vi "Auto_Routine_QuickAuto.vi"(8 "error in (no error)":errorcluster, 9 "Distance(Back)":dbl, 10 "Game Piece":T1, 11 "Position":T2=enum."Middle") -> (0 "error out":errorcluster)   [LabVIEW 2020]
uses:
  Arm/ArmPositionPreset.ctl
  Arm/ArmGamePiecePreset.ctl
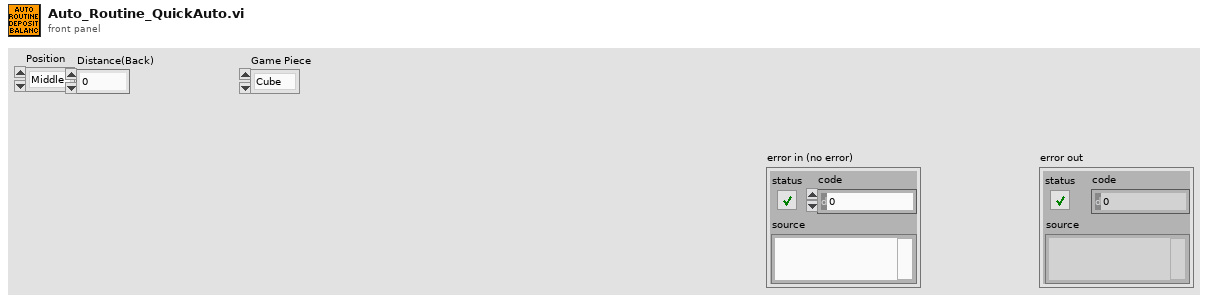
[diagram p1: front panel]
types:
  T1 = typedef "ArmGamePiecePreset.ctl" = enum16{"Cube", "Cone"}
  T2 = typedef "ArmPositionPreset.ctl" = enum16{"Upper", "Lower", "Middle", "Home", "Shelf", "Floor"}
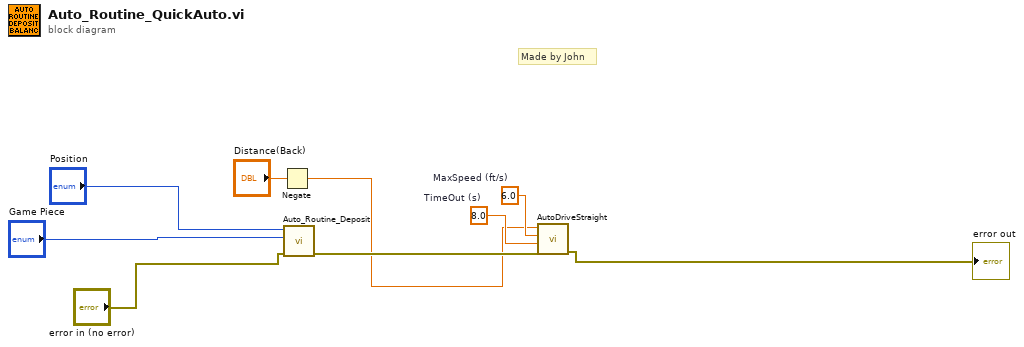
[diagram p0: block diagram]
diagram:
  w7 = 8.0  # TimeOut (s)
  w8 = 6.0  # MaxSpeed (ft/s)
  # "Made by John"
  n1 = Negate(x="Distance(Back)") -> (-x=w2:dbl)
  n2 = call "Auto_Routine_Deposit.vi"("error in (no error)"="error in (no error)", "Game Piece"="Game Piece", "Position"="Position") -> ("error out"=w9:errorcluster)  [unwired: 8 in]
  n3 = call "AutoDriveStraight.vi"("error in (no error)"=w9, "TimeOut (s)"=w7, "MaxSpeed (ft/s)"=w8, "Dist (ft)"=w2) -> ("error out"=→"error out":errorcluster)  [unwired: 7 in]
